vi "_io_read_bin_data_instrument_to_PC.vi"(7 "Direct Block Size in (Read and parse)":i64=-1, 8 "error in":errorcluster caption="error in (no error)", 11 "VISA resource name":refnum<visa-resource-name>) -> (0 "error out":errorcluster, 1 "Data size Int64":i32, 2 "Data out":string, 3 "VISA resource name out":refnum<visa-resource-name>)   [LabVIEW 2020, in "Rohde&Schwarz RTx Oscilloscopes.lvlib" / "rsidr_core.lvlib"]
uses:
  rsidr_core.lvlib
  type_Error_Codes.ctl
  type_AdditionalFlag_Bits.ctl
  _type_Operation_Fgv_Debug.ctl
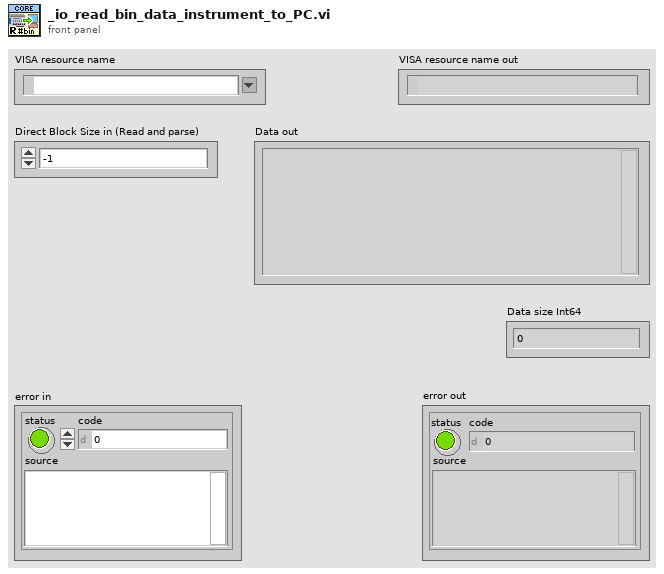
[diagram p1: front panel]
types:
  T1 = typedef "Rohde&Schwarz RTx Oscilloscopes.lvlib/rsidr_core.lvlib/type_Error_Codes.ctl" = enum16{"No_error", "VISA_err_ResourceNotFound", "VISA_err_Timeout", "VISA_warn_MoreDataAvailable", "RS_err_MissingCallback", "RS_err_InvalidAttribute", "RS_err_InvalidValue", "RS_err_UnknownResource", "RS_err_AlreadyInitialized", "RS_err_InstrumentStatus", "RS_err_BadRepCapName", "RS_err_TypesMismatch", "RS_err_ValueNotSupported", "RS_err_InvalidRngTable", "RS_err_IDqueryFail", "RS_err_UnexpResponse", "VISA_warn_ConfigNotLoaded", "RS_err_AttributeNotReadable", "RS_err_AttributeNotWritable", "RS_err_InstrumentType", "RS_err_InstrumentOption", "VISA_err_InvalidSize", "RS_err_ReliabilityIndicator", "VISA_warn_UnknownStatus", "VISA_warn_TermCharRead", "VISA_err_IO_error", "RS_err_FunctionNotSupported", "VISA_warn_QueueEmpty"}
  T2 = typedef "Rohde&Schwarz RTx Oscilloscopes.lvlib/rsidr_core.lvlib/type_AdditionalFlag_Bits.ctl" = enum16{"Send LF after Bin Block", "Junk read with io_clear_buffers.vi", "io_clear_buffers: viClear()", "io_clear_buffers: viFlush()", "<NotUsed1>", "Allow Dbl & Int Bin/Ascii read", "*OPC? in check_instrument_error.vi", "<NotUsed2>", "Smart Enum Matching", "Less Strict RepCaps check", "AssureResponseEndWithLF"}
  T3 = typedef "Rohde&Schwarz RTx Oscilloscopes.lvlib/rsidr_core.lvlib/_type_Operation_Fgv_Debug.ctl" = enum16{"Reset", "ReadCommand", "SetCommand"}
  T4 = typedef "Rohde&Schwarz RTx Oscilloscopes.lvlib/rsidr_core.lvlib/type_Session_Data.ctl" = cluster{"IDN string":string, "Instrument FW":string, "Instr type":string, "Instr type for err. msg.":string, "Installed Options":string[], "Ignore Error Messages":string, "Logging params":variant, "OPC Timeout":i32, "VISA Timeout":i32, "STB Poll VISA Timeout":i32, "Additional Flags":i32, "Wait Before Read":i32, "Wait Before Write":i32, "Option String Flags":i32, "IO Segment Size":i64, "VISA Access Mode":T5, "Interface Type":T6, "OPC Wait Mode":T7, "Bin Float Number  Format":T8, "Bin Integer Number Format":T9, "Simulate":bool, "VXIcapable":bool, "Duplicate Session":bool, "Add LF to Write":bool, "Logging":bool, "Fast Sweep":bool, "Query Instrument Status":bool, "Check Range":bool, "Check Options":bool, "OPC-sync Attr Writes":bool, "OPC-sync Attr Queries":bool}
  T5 = typedef "Rohde&Schwarz RTx Oscilloscopes.lvlib/rsidr_core.lvlib/type_VisaAccessMode.ctl" = u16
  T6 = typedef "Rohde&Schwarz RTx Oscilloscopes.lvlib/rsidr_core.lvlib/type_InterfaceType.ctl" = enum16{"Unknown", "GPIB", "VXI", "GPIB_VXI", "ASRL", "PXI", "TCPIP", "USB", "SOCKET"}
  T7 = typedef "Rohde&Schwarz RTx Oscilloscopes.lvlib/rsidr_core.lvlib/type_OPC_Wait_Mode.ctl" = enum16{"STBpolling", "STBpollingSlow", "STBpollingSuperSlow", "ServiceRequest", "OPCquery"}
  T8 = typedef "Rohde&Schwarz RTx Oscilloscopes.lvlib/rsidr_core.lvlib/type_Binary_Float_Number_Format.ctl" = enum16{"Float_4_Bytes_Swapped", "Float_4_Bytes", "Double_8_Bytes_Swapped", "Double_8_Bytes"}
  T9 = typedef "Rohde&Schwarz RTx Oscilloscopes.lvlib/rsidr_core.lvlib/type_Binary_Integer_Number_Format.ctl" = enum16{"Int32_4_Bytes_Swapped", "Int32_4 Bytes", "Int16_2_Bytes_Swapped", "Int16_2_Bytes"}
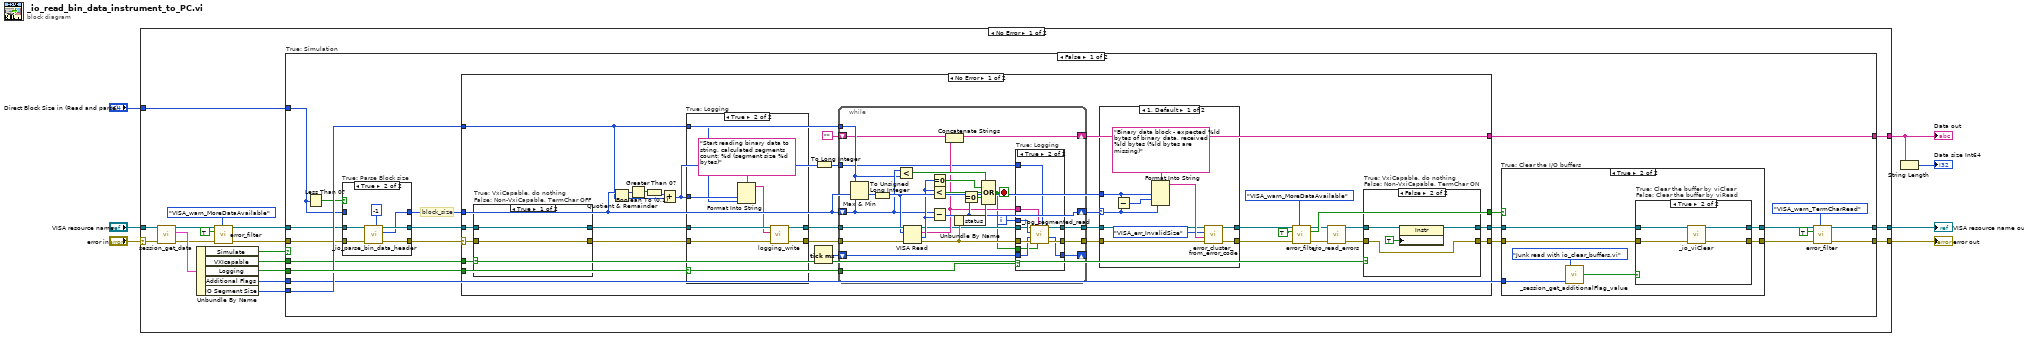
[diagram p0: block diagram]
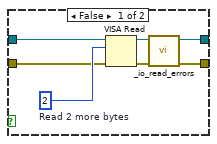
[diagram p4: hidden frame]
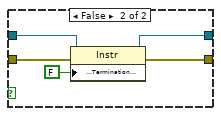
[diagram p6: hidden frame]
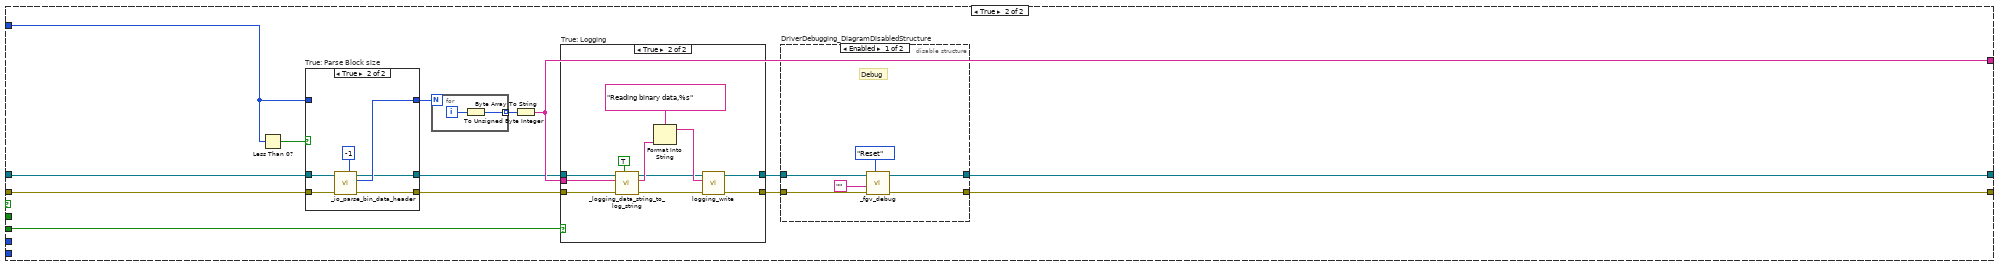
[diagram p11: hidden frame]
diagram:
  n1 = case shown="No Error" "error in" {
    selector: "error in" -> [w23 w232]
    tunnel: [w25 w231] -> w7
    tunnel: [w24 w232] -> w6
    tunnel: "VISA resource name" -> [w22 w231]
    tunnel: [w18 _] -> w3
    tunnel: "Direct Block Size in (Read and parse)" -> [w14 _]
    frame No Error {
      n2 = call "session_get_data.vi"("error in"=w23, "VISA resource name"=w22) -> ("error out"=w11:errorcluster, "Session User Data out"=w20:T4, "VISA resource name out"=w10:refnum<visa-resource-name>)  [unwired: 6 in, 1 out]
      n3 = Unbundle By Name(w20) -> ("Simulate"=w21:bool, "VXIcapable"=w19:bool, "Logging"=w17:bool, "Additional Flags"=w16:i32, "IO Segment Size"=w15:i64)
      n4 = call "error_filter.vi"("Error Enum in"=type_Error_Codes."VISA_warn_MoreDataAvailable", "error in"=w11, "Clear detected code (F)"=TRUE, "VISA resource name"=w10) -> ("error out"=w9:errorcluster, "VISA resource name out"=w8:refnum<visa-resource-name>)  [unwired: 5 in, 1 out]
      n5 = case "True: Simulation" shown="False" w21 {
        tunnel: w9 -> [w29 w190]
        tunnel: w8 -> [w30 w189]
        tunnel: [w35 w197] -> w25
        tunnel: [w34 w198] -> w24
        tunnel: w19 -> [w28 _]
        tunnel: [w43 w192] -> w18
        tunnel: w17 -> [w42 w193]
        tunnel: w15 -> [w41 _]
        tunnel: w16 -> [w40 _]
        tunnel: w14 -> [w32 w186]
        frame False {
          # "block_size"
          n6 = Less Than 0?(x=w32) -> (x < 0?=w33:bool)
          n7 = case "True: Parse Block size" shown="True" w33 {
            tunnel: w29 -> [w47 w55]
            tunnel: w30 -> [w49 w54]
            tunnel: [w47 w53] -> w46
            tunnel: [w49 w52] -> w45
            tunnel: [w48 w51] -> w44
            tunnel: w32 -> [w48 _]
            frame False {
            }
            frame True {
              n8 = call "_io_parse_bin_data_header.vi"("Timeout for chunked touts"=-1 ("Timeout for long reads (-1: No long reads)"), "error in"=w55, "VISA resource name"=w54) -> ("error out"=w53:errorcluster, "Size of the bin data"=w51:i64, "VISA resource name out"=w52:refnum<visa-resource-name>)  [unwired: 4 in, 2 out]
            }
          }
          n9 = case shown="No Error" w46 {
            selector: w46 -> [w81 w184]
            tunnel: [w77 w184] -> w27
            tunnel: w45 -> [w84 w183]
            tunnel: w44 -> [w88 _]
            tunnel: w41 -> [w87 _]
            tunnel: [w78 w183] -> w26
            tunnel: [w108 _] -> w43
            tunnel: w42 -> [w95 _]
            tunnel: [w97 _] -> w31
            tunnel: w28 -> [w76 _]
            frame No Error {
              n10 = case "True: VxiCapable, do nothing\nFalse: Non-VxiCapable, TermChar OFF" shown="True" w76 {
                tunnel: w81 -> [w115 w121]
                tunnel: w84 -> [w116 w120]
                tunnel: [w116 w119] -> w83
                tunnel: [w115 w118] -> w82
                frame True {
                }
                frame False {
                  n11 = property on="Property Node" class="Instr"(reference=w120, error in=w121, "Message Based Settings:Termination Character Enable"=FALSE ("TermChar En")) -> (reference out=w119:refnum<visa-resource-name>, error out=w118:errorcluster)
                }
              }
              n12 = Quotient & Remainder(x=w88, y=w87) -> (x-y*floor(x/y)=w91:i64, floor(x/y)=w92:i64)
              n13 = Greater Than 0?(x=w91) -> (x > 0?=w90:bool)
              n14 = Boolean To (0,1)(Boolean=w90) -> (0, 1=w89:i16)
              n15 = Add(x=w89, y=w92) -> (x+y=w86:i64)
              n16 = case "True: Logging" shown="True" w95 {
                tunnel: w82 -> [w174 w180]
                tunnel: [w174 w182] -> w102
                tunnel: w83 -> [w173 w179]
                tunnel: [w173 w181] -> w103
                tunnel: w87 -> [_ w175]
                tunnel: w86 -> [_ w176]
                frame False {
                }
                frame True {
                  n17 = Format Into String(format string="Start reading binary data to string, calculated segments count: %d (segment size %d bytes)", w176, w175) -> (resulting string=w177:string)  [unwired: 2 in, 1 out]
                  n18 = call "logging_write.vi"("error in"=w180, "String to write"=w177, "VISA resource name"=w179) -> ("error out"=w182:errorcluster, "VISA resource name out"=w181:refnum<visa-resource-name>)  [unwired: 7 in]
                }
              }
              n19 = Tick Count (ms)() -> (millisecond timer value=w96:u32)
              n20 = To Long Integer(number=w86) -> (32bit integer=w85:i32)
              n21 = while {
                tunnel: w102 -> [w145]
                tunnel: w103 -> [w147]
                tunnel: w87 -> [w139]
                shift-right: [w133] -> w104
                shift-left: w88 -> [w140]
                tunnel: [w130] -> w105
                shift-right: [w137] -> w108
                shift-left: "" ("Empty String Constant") -> [w136]
                tunnel: [w124] -> w107
                shift-right: [w128] -> _
                shift-left: w96 -> [w129]
                tunnel: w95 -> [w131]
                tunnel: w85 -> [w123]
                i -> [w127]
                stop <- w122 stop-if-true
                n22 = Max & Min(x=w139, y=w140) -> (min(x,y)=w146:i64)  [unwired: 1 out]
                n23 = To Unsigned Long Integer(number=w146) -> (unsigned 32bit integer=w144:u32)
                n24 = Less?(x=w140, y=w139) -> (x < y?=w138:bool)
                n25 = VISA Read(VISA resource name=w147, byte count=w144, error in (no error)=w145) -> (VISA resource name out=w125:refnum<visa-resource-name>, read buffer=w126:string, return count=w143:u32, error out=w132:errorcluster)
                n26 = Equal To 0?(x=w143) -> (x = 0?=w141:bool)
                n27 = Less?(x=w143, y=w144) -> (x < y?=w142:bool)
                n28 = Subtract(x=w140, y=w143) -> (x-y=w133:i64)
                n29 = Concatenate Strings(w136, w126) -> (w137:string)
                n30 = Unbundle By Name(w132) -> ("status"=w135:bool)
                n31 = Equal To 0?(x=w133) -> (x = 0?=w134:bool)
                n32 = Compound Arithmetic op=OR(w138, w141, w142, w134, w135) -> (w122:bool)
                n33 = case "True: Logging" shown="True" w131 {
                  tunnel: w132 -> [w150 w160]
                  tunnel: [w150 w159] -> w130
                  tunnel: w129 -> [w149 w158]
                  tunnel: [w149 w157] -> w128
                  tunnel: w127 -> [_ w156]
                  tunnel: w126 -> [_ w155]
                  tunnel: w125 -> [w148 w154]
                  tunnel: [w148 w153] -> w124
                  tunnel: w123 -> [_ w152]
                  tunnel: w122 -> [_ w151]
                  frame False {
                  }
                  frame True {
                    n34 = call "_log_segmented_read.vi"("Total Segments"=w152, "Last Segment"=w151, "Data"=w155, "error in"=w160, "Previous Start Time ms"=w158, "Segment Ix"=w156, "VISA resource name"=w154) -> ("error out"=w159:errorcluster, "New Start Time ms"=w157:u32, "VISA resource name out"=w153:refnum<visa-resource-name>)  [unwired: 2 in]
                  }
                }
              }
              n35 = case shown="1, Default" w104 {
                selector: w104 -> [w165 _]
                tunnel: w105 -> [w168 w172]
                tunnel: [w169 w172] -> w99
                tunnel: w88 -> [w167 _]
                tunnel: w107 -> [w162 w171]
                tunnel: [w161 w171] -> w98
                frame 1, Default {
                  n36 = Subtract(x=w167, y=w165) -> (x-y=w166:i64)
                  n37 = Format Into String(format string="Binary data block - expected %ld bytes of binary data, received %ld bytes (%ld bytes are missing)" ("error message (\"\")"), w167, w166, w165) -> (resulting string=w164:string)  [unwired: 2 in, 1 out]
                  n38 = call "error_cluster_from_error_code.vi"("error in"=w168, "Error Message (\"\")"=w164, "Error Enum in"=type_Error_Codes."VISA_err_InvalidSize", "VISA resource name"=w162) -> ("error out"=w169:errorcluster, "VISA resource name out"=w161:refnum<visa-resource-name>)  [unwired: 6 in]
                }
                frame 0 {
                }
              }
              n39 = call "error_filter.vi"("Error Enum in"=type_Error_Codes."VISA_warn_MoreDataAvailable" ("Code to detect"), "error in"=w99, "Clear detected code (F)"=TRUE ("Clear detected error (F)"), "VISA resource name"=w98) -> ("error out"=w93:errorcluster, "Code Detected"=w97:bool, "VISA resource name out"=w94:refnum<visa-resource-name>)  [unwired: 5 in]
              n40 = call "_io_read_errors.vi"("error in"=w93, "VISA resource name"=w94) -> ("error out"=w79:errorcluster, "VISA resource name out"=w80:refnum<visa-resource-name>)  [unwired: 8 in]
              n41 = case "True: VxiCapable, do nothing\nFalse: Non-VxiCapable, TermChar ON" shown="False" w76 {
                tunnel: w80 -> [w110 w114]
                tunnel: [w110 w113] -> w78
                tunnel: w79 -> [w109 w112]
                tunnel: [w109 w112] -> w77
                frame True {
                }
                frame False {
                  n42 = property on="Property Node" class="Instr"(reference=w114, "Message Based Settings:Termination Character Enable"=TRUE) -> (reference out=w113:refnum<visa-resource-name>)  [unwired: 1 in, 1 out]
                }
              }
            }
            frame Error {
            }
          }
          n43 = case "True: Clear the I/O buffers" shown="True" w31 {
            tunnel: [w56 w62] -> w36
            tunnel: w26 -> [w57 w63]
            tunnel: w27 -> [w56 w64]
            tunnel: [w57 w61] -> w37
            tunnel: w40 -> [_ w59]
            frame False {
            }
            frame True {
              n44 = call "_session_get_additionalFlag_value.vi"("AdditionalFlags value in"=w59, "AdditionalFlag bit"=type_AdditionalFlag_Bits."Junk read with io_clear_buffers.vi") -> ("AdditionalFlag bit value out"=w60:bool)  [unwired: 3 in]
              n45 = case "True: Clear the buffer by viClear\nFalse: Clear the buffer by viRead" shown="True" w60 {
                tunnel: w64 -> [w65 w75]
                tunnel: w63 -> [w66 w74]
                tunnel: [w69 w73] -> w62
                tunnel: [w68 w72] -> w61
                frame False {
                  w67 = u32 2  # Read 2 more bytes
                  n46 = VISA Read ("Read the junk")(VISA resource name=w66, byte count=w67, error in (no error)=w65) -> (VISA resource name out=w70:refnum<visa-resource-name>, error out=w71:errorcluster)  [unwired: 2 out]
                  n47 = call "_io_read_errors.vi"("error in"=w71, "VISA resource name"=w70) -> ("error out"=w69:errorcluster, "VISA resource name out"=w68:refnum<visa-resource-name>)  [unwired: 8 in]
                }
                frame True {
                  n48 = call "_io_viClear.vi"("error in"=w75, "VISA resource name"=w74) -> ("error out"=w73:errorcluster, "VISA resource name out"=w72:refnum<visa-resource-name>)  [unwired: 8 in]
                }
              }
            }
          }
          n49 = call "error_filter.vi"("Error Enum in"=type_Error_Codes."VISA_warn_TermCharRead", "error in"=w36, "Clear detected code (F)"=TRUE, "VISA resource name"=w37) -> ("error out"=w34:errorcluster, "VISA resource name out"=w35:refnum<visa-resource-name>)  [unwired: 5 in, 1 out]
        }
        frame True {
          n50 = Less Than 0?(x=w186) -> (x < 0?=w191:bool)
          n51 = case "True: Parse Block size" shown="True" w191 {
            tunnel: w190 -> [w199 w206]
            tunnel: w189 -> [w201 w205]
            tunnel: [w199 w204] -> w188
            tunnel: [w201 w203] -> w187
            tunnel: [w200 w207] -> w185
            tunnel: w186 -> [w200 _]
            frame False {
            }
            frame True {
              n52 = call "_io_parse_bin_data_header.vi"("Timeout for chunked touts"=-1 ("Timeout for long reads (-1: No long reads)"), "error in"=w206, "VISA resource name"=w205) -> ("error out"=w204:errorcluster, "Size of the bin data"=w207:i64, "VISA resource name out"=w203:refnum<visa-resource-name>)  [unwired: 4 in, 2 out]
            }
          }
          n53 = for {
            N: w185 -> [_]
            tunnel: [w221] -> w196 mode=indexing
            i -> [w222]
            n54 = To Unsigned Byte Integer(number=w222) -> (unsigned 8bit integer=w221:u8)
          }
          n55 = Byte Array To String(unsigned byte array=w196) -> (string=w192:string)
          n56 = case "True: Logging" shown="True" w193 {
            tunnel: w188 -> [w209 w215]
            tunnel: [w209 w210] -> w194
            tunnel: w187 -> [w208 w214]
            tunnel: [w208 w211] -> w195
            tunnel: w192 -> [_ w217]
            frame False {
            }
            frame True {
              n57 = call "_logging_data_string_to_log_string.vi"("Force binary format (F)"=TRUE, "error in"=w215, "Raw string to log"=w217, "VISA resource name"=w214) -> ("error out"=w213:errorcluster, "Result log string"=w218:string, "VISA resource name out"=w212:refnum<visa-resource-name>)  [unwired: 5 in]
              n58 = Format Into String(format string="Reading binary data,%s", w218) -> (resulting string=w219:string)  [unwired: 2 in, 1 out]
              n59 = call "logging_write.vi"("error in"=w213, "String to write"=w219, "VISA resource name"=w212) -> ("error out"=w210:errorcluster, "VISA resource name out"=w211:refnum<visa-resource-name>)  [unwired: 7 in]
            }
          }
          n60 = disable-structure "DriverDebugging_DiagramDisabledStructure" shown="Enabled" {
            disable-tunnel: w194 -> [w228 w229]
            disable-tunnel: [w226 w229] -> w198
            disable-tunnel: w195 -> [w227 w230]
            disable-tunnel: [w225 w230] -> w197
            frame Enabled {
              # "Debug"
              n61 = call "_fgv_debug.vi"("Operation"=_type_Operation_Fgv_Debug."Reset", "error in"=w228, "Command in"="" ("Empty String Constant"), "VISA resource name"=w227) -> ("error out"=w226:errorcluster, "VISA resource name out"=w225:refnum<visa-resource-name>)  [unwired: 6 in]
            }
            frame Disabled {
              # "Release"
            }
          }
        }
      }
    }
    frame Error {
    }
  }
  "error out" <- w6
  "VISA resource name out" <- w7
  "Data out" <- w3
  n62 = String Length(string=w3) -> (length=→"Data size Int64":i32)
